vi "MotionProfileTesting.vi"() -> ()   [LabVIEW 2016]
panel:
  in  "Go":bool
  in  "Go Backwards":bool
  out "Vel":cluster{dbl, "vel":dbl}(graph)
  out "Pos":cluster{dbl, "pos":dbl}(graph)={50.0, "pos"=48.31556625}
  in  "Linear Constants":T1={"FF"=0.009, "AFF"=0.002, "PID gains"={"P"=0.07, "I"=0.0, "D"=0.0}} {"PID gains"."D" format="%.3f"; "PID gains"."I" format="%.3f"; "PID gains"."P" format="%.3f"}
  in  "Distance":dbl=50.0
  in  "InitialVelocity":dbl
  in  "FinalVelocity":dbl
  in  "MaxVelocity":dbl=50.0
  in  "MaxAccel":dbl=30.0
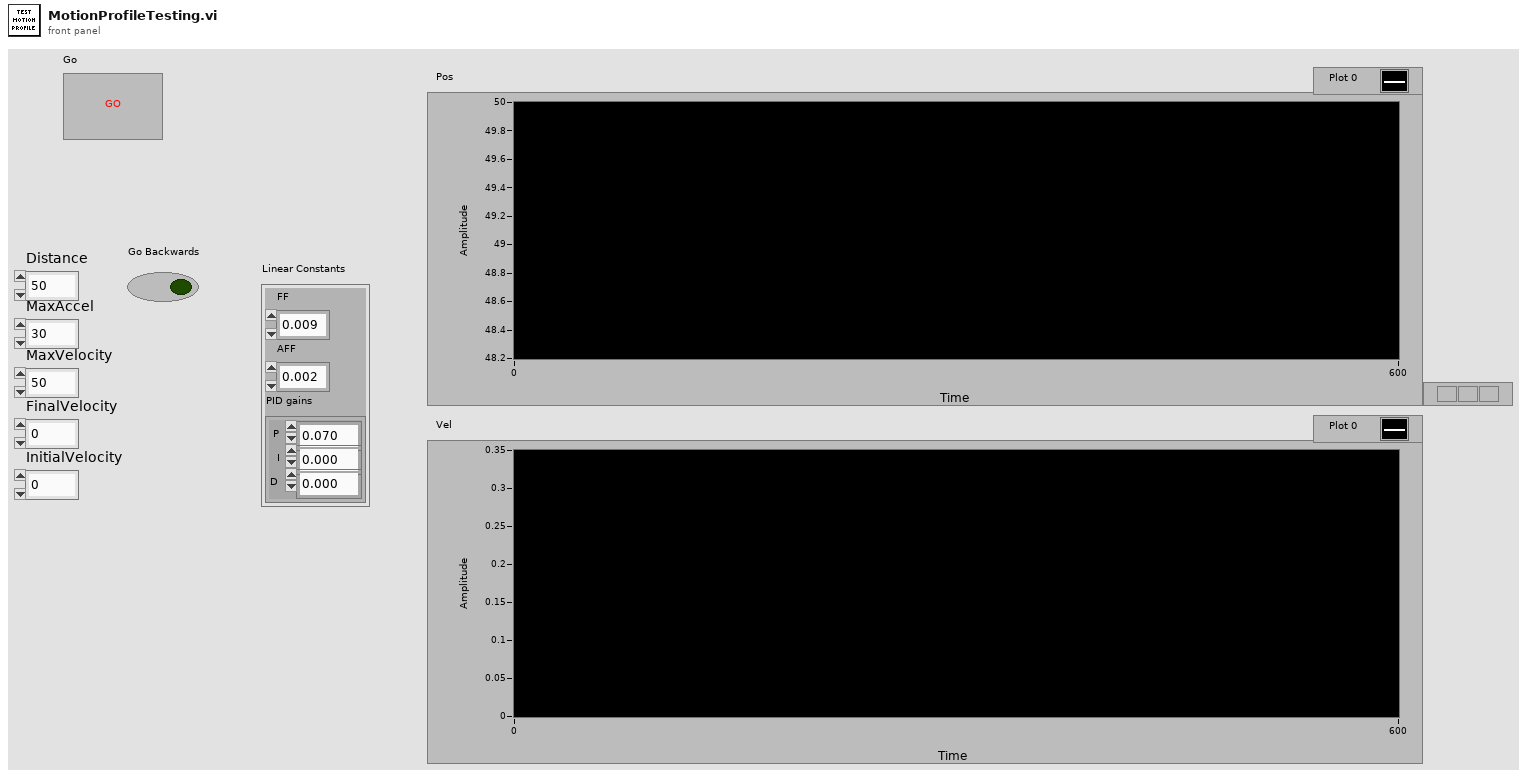
[diagram p1: front panel]
types:
  T1 = cluster{"FF":dbl, "AFF":dbl, "PID gains":cluster{"P":dbl, "I":dbl, "D":dbl}}
  T2 = cluster{dbl, "distance/rotation":dbl, "distance/rotation":dbl}
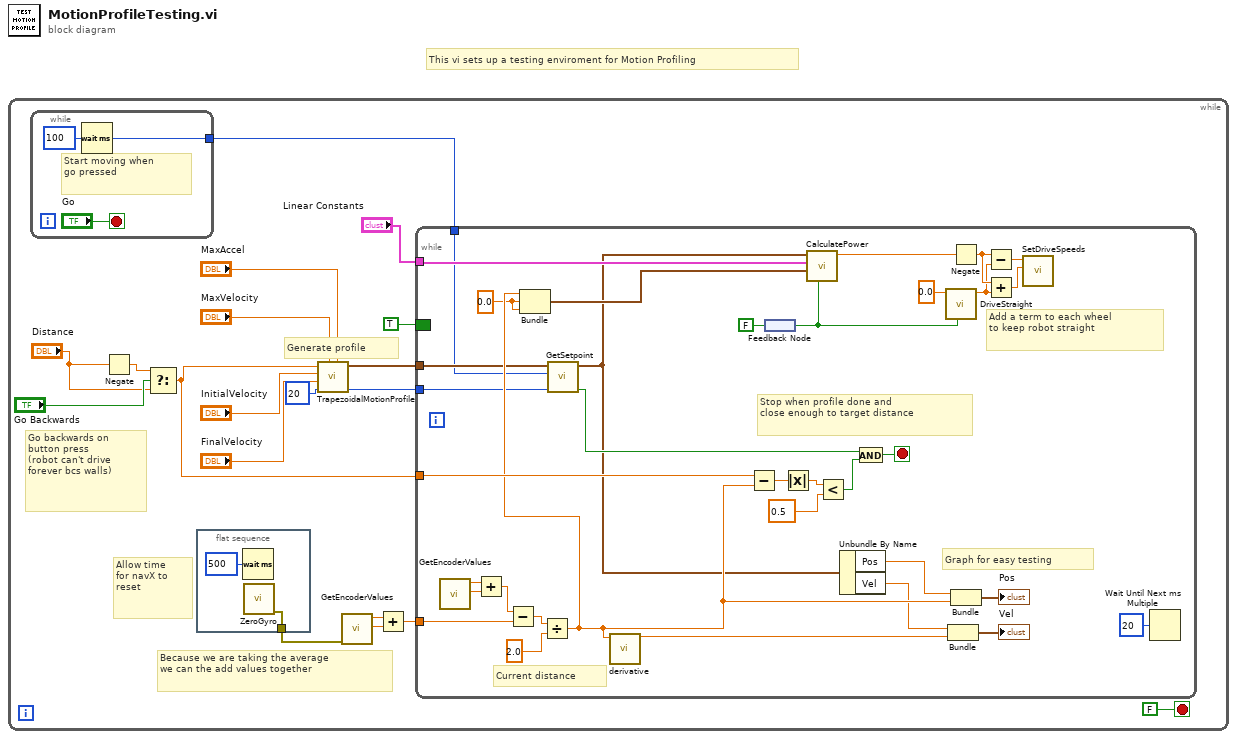
[diagram p0: block diagram]
diagram:
  # "This vi sets up a testing enviroment for Motion Profiling"
  n1 = while {
    stop <- FALSE stop-if-true
    # "Go backwards on\nbutton press\n(robot can't drive\nforever bcs walls)"
    # "Allow time\nfor navX to\nreset"
    # "Because we are taking the average\nwe can the add values together"
    # "Generate profile"
    n2 = while {
      tunnel: [w22] -> w3
      stop <- "Go" stop-if-true
      # "Start moving when\ngo pressed"
      n3 = Wait (ms)(milliseconds to wait=u32 100 ("millisecond multiple")) -> (millisecond timer value=w22:u32)
    }
    n4 = Negate(x="Distance") -> (-x=w11:dbl)
    n5 = Select(t=w11, s="Go Backwards", f="Distance") -> (s? t:f=w9:dbl)
    n6 = flat-sequence {
      tunnel: [w20] -> w4
      frame #0 {
        n7 = Wait (ms)(milliseconds to wait=u32 500 ("millisecond multiple")) -> ()  [unwired: 1 out]
        n8 = call "ZeroGyro.vi"() -> ("error out"=w20:errorcluster)  [unwired: 11 in]
      }
    }
    n9 = call "TrapezoidalMotionProfile.vi"("MaxAccel"="MaxAccel", "MaxVelocity"="MaxVelocity", "dt"=u32 20, "FinalVelocity"="FinalVelocity", "InitialVelocity"="InitialVelocity", "Distance"=w9) -> ("dt"=w1:u32, "Profile"=w15:cluster{"Pos":dbl, "Vel":dbl, "Accel":dbl}[])  [unwired: 4 in]
    n10 = call "GetEncoderValues.vi"("error in"=w4) -> ("RightDistance"=w6:dbl, "LeftDistance"=w7:dbl)  [unwired: 8 in, 1 out]
    n11 = Add(x=w7, y=w6) -> (x+y=w5:dbl)
    n12 = while {
      tunnel: w15 -> [w34]
      tunnel: "Linear Constants" -> [w41]
      tunnel: w9 -> [w50]
      border: TRUE ("Reset") -> [_]
      tunnel: w5 -> [w44]
      tunnel: w3 -> [w32]
      tunnel: w1 -> [w33]
      stop <- w51 stop-if-true
      w38 = 0.0 ("distance/rotation")
      # "Add a term to each wheel\nto keep robot straight"
      # "Stop when profile done and\nclose enough to target distance"
      # "Graph for easy testing"
      # "Current distance"
      n13 = call "GetEncoderValues.vi"() -> ("RightDistance"=w48:dbl, "LeftDistance"=w47:dbl)  [unwired: 9 in, 1 out]
      n14 = Add(x=w47, y=w48) -> (x+y=w45:dbl)
      n15 = Subtract(x=w45, y=w44) -> (x-y=w46:dbl)
      n16 = Divide(x=w46, y=2.0 ("distance/rotation")) -> (x/y=w39:dbl)
      n17 = Bundle(w39, "distance/rotation"=w38, "distance/rotation"=w38) -> (w40:T2)  [unwired: 1 in]
      n18 = call "GetSetpoint.vi"("dt"=w33, "Start Time"=w32, "Profile"=w34) -> ("Profile done?"=w31:bool, "Setpoints"=w30:cluster{"Pos":dbl, "Vel":dbl, "Accel":dbl})  [unwired: 7 in]
      n19 = call "derivative.vi"("x"=w39) -> ("dx/dt"=w49:dbl)  [unwired: 10 in]
      n20 = Subtract(x=w50, y=w39) -> (x-y=w57:dbl)
      n21 = feedback-in #1(FALSE ("Reset")) -> ()
      n22 = feedback #1() -> (w25:bool)
      n23 = Absolute Value(x=w57) -> (abs(x)=w56:dbl)
      n24 = call "CalculatePower.vi"("Reset"=w25, "Process Variables"=w40, "Constants"=w41, "Setpoints"=w30) -> ("Power"=w37:dbl)  [unwired: 7 in]
      n25 = Less?(x=w56, y=0.5 ("Closeness at end")) -> (x < y?=w36:bool)
      n26 = Unbundle By Name(w30) -> ("Pos"=w29:dbl, "Vel"=w28:dbl)
      n27 = And(x=w31, y=w36) -> (x .and. y?=w51:bool)
      n28 = call "DriveStraight.vi"("Reset"=w25, "Angle"=0.0) -> ("Turn"=w53:dbl)  [unwired: 9 in]
      n29 = Bundle("Vel"=w28, "dx/dt"=w49) -> (→"Vel":cluster{"Vel":dbl, "dx/dt":dbl})  [unwired: 1 in]
      n30 = Negate(x=w37) -> (-x=w54:dbl)
      n31 = Bundle("Pos"=w29, w39) -> (→"Pos":cluster{"Pos":dbl, dbl})  [unwired: 1 in]
      n32 = Subtract(x=w54, y=w53) -> (x-y=w43:dbl)
      n33 = Add(x=w54, y=w53) -> (x+y=w42:dbl)
      n34 = call "SetDriveSpeeds.vi"("Right Value"=w42, "Left Value"=w43) -> ()  [unwired: 9 in, 1 out]
      n35 = Wait Until Next ms Multiple(millisecond multiple=u32 20) -> ()  [unwired: 1 out]
    }
  }
